vi "releaseany.vi"(8 "error in":errorcluster, 9 "buffer size":u64, 11 "Buffers":T1[](array[typedef])) -> (0 "error out":errorcluster, 1 "is locked":bool, 2 "output buffer":T1, 3 "Buffers out":T1[](array[typedef]))   [LabVIEW 2016]
uses:
  private/vis/BufferStruct.ctl
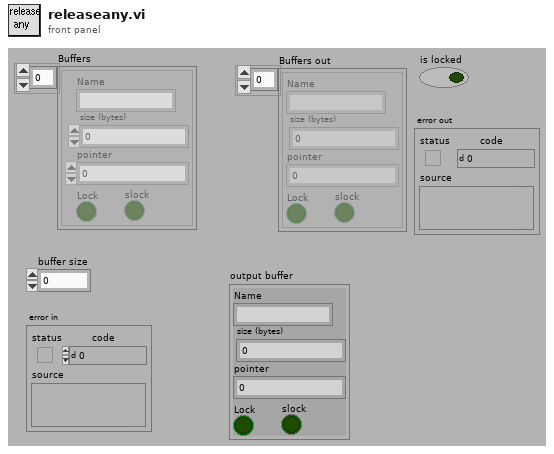
[diagram p1: front panel]
types:
  T1 = typedef "BufferStruct.ctl" = cluster{"Name":string, "size (bytes)":u64, "pointer":u64, "Lock":bool, "slock":bool}
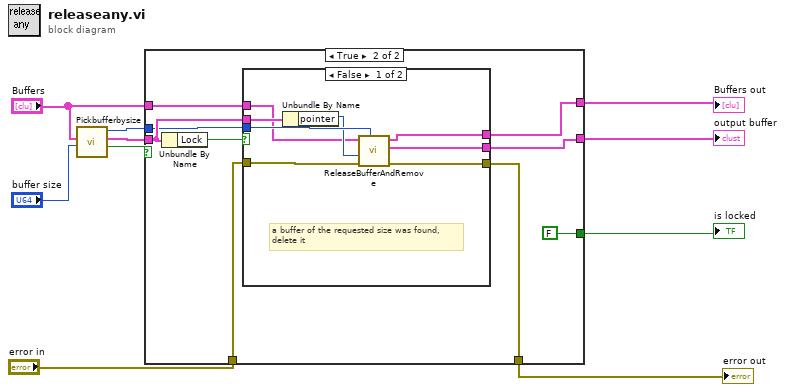
[diagram p0: block diagram]
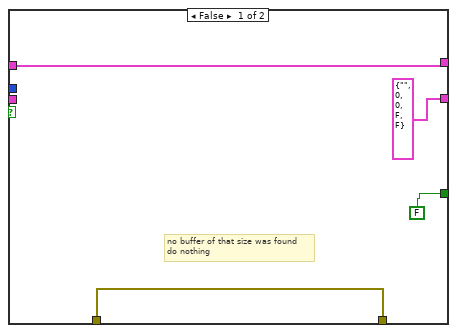
[diagram p2: hidden frame]
diagram:
  n1 = call "Pickbufferbysize.vi"("buffer size"="buffer size", "Buffers"="Buffers") -> ("found"=w3:bool, "buffer found"=w4:T1, "index"=w10:i32)  [unwired: 7 out]
  n2 = case shown="True" w3 {
    tunnel: w4 -> [_ w18]
    tunnel: [T1 {"Name"="", "size (bytes)"=0, "pointer"=0, "Lock"=FALSE, "slock"=FALSE} ("buffer found") w21] -> w5
    tunnel: "error in" -> [w13 w23]
    tunnel: [w13 w22] -> w7
    tunnel: [w11 w15] -> w8
    tunnel: [FALSE ("Lock") FALSE ("Lock")] -> w9
    tunnel: w10 -> [_ w17]
    tunnel: "Buffers" -> [w11 w16]
    frame False {
      # "no buffer of that size was found\ndo nothing"
    }
    frame True {
      n3 = Unbundle By Name(w18) -> ("Lock"=w19:bool)
      n4 = case shown="False" w19 {
        tunnel: w23 -> [w31 w33]
        tunnel: [w30 w33] -> w22
        tunnel: [w29 w34] -> w21
        tunnel: w18 -> [w27 w34]
        tunnel: w17 -> [w28 _]
        tunnel: w16 -> [w25 w32]
        tunnel: [w24 w32] -> w15
        frame False {
          # "a buffer of the requested size was found,\ndelete it"
          n5 = Unbundle By Name(w27) -> ("pointer"=w26:u64)
          n6 = call "ReleaseBufferAndRemove.vi"("index"=w28, "error in (no error)"=w31, "pointer"=w26, "Buffers"=w25) -> ("error out"=w30:errorcluster, "output buffer"=w29:T1, "output buffers"=w24:T1[])  [unwired: 1 in, 4 out]
        }
        frame True {
          # "a buffer of the requested size was found,\nbut is locked. Do nothing"
        }
      }
    }
  }
  "is locked" <- w9
  "Buffers out" <- w8
  "error out" <- w7
  "output buffer" <- w5
